vi "IdentifyBlob_Square_Cluster.vi"(1 "color":u32(colorbox)=16773418, 2 "Centroid":cluster{"X":dbl, "Y":dbl}, 3 "Dimension":i32=20, 4 "Image in":T1 {"Dialogs" format="%.0b"}) -> (0 "picture":picture)   [LabVIEW 2024]
doc: "This VI is used with the BlobTracking.vi or the BiggestComplexBlob.vi. It will draw a shape centered on the blob's centroid. The shape depends upon the shape chosen by the poly selector and the dimension wired to the VI."
uses:
  <userlib>/ImageProcessing/QTLIB_2595_LV86/QT_Image.ctl
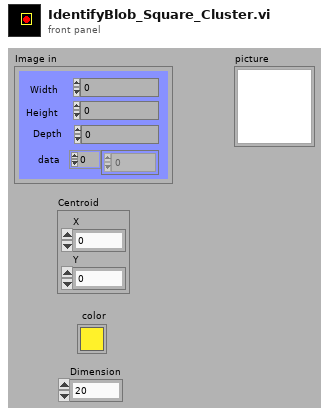
[diagram p1: front panel]
types:
  T1 = typedef "QT_Image.ctl" = cluster{"Width":i32, "Height":i32, "Depth":i32, "data":u8[], "Compressed data":u8[], "Color table":u32[], "Duration":i32, "Options":i32, "Timestamp":i32, "ID":i32, "Reserved":i32, "Dialogs":u32}
  T2 = cluster{"left":i16, "top":i16, "right":i16, "bottom":i16}
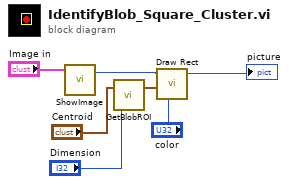
[diagram p0: block diagram]
diagram:
  n1 = call <userlib>:"ShowImage.vi"("Image"="Image in") -> ("image"=w3:picture)  [unwired: 2 in, 1 out]
  n2 = call <userlib>:"GetBlobROI.vi"("Dimension"="Dimension", "Centroid"="Centroid") -> ("ROI"=w2:T2)  [unwired: 1 out]
  n3 = call <vilib>:"Draw Rect.vi"("picture"=w3, "rect"=w2, "color(black)"="color") -> ("new picture"=→"picture":picture)  [unwired: 6 in]
